vi "Signal in Single Point.vi"() -> ()   [LabVIEW 2025]
uses:
  <vilib>/xnet/xnet.llb/XNET Create Session (Signal Input Single-point).vi
  <vilib>/xnet/xnet.llb/XNET Read (Signal Single-point).vi
panel:
  out "Barra":dbl(graph)
  out "Abs":dbl(graph)
  in  "signal list":refnum<k21>[](array[refnum])
  in  "Wait":u32=200
  in  "stop":bool
  in  "interface":refnum<k21>="CAN1"
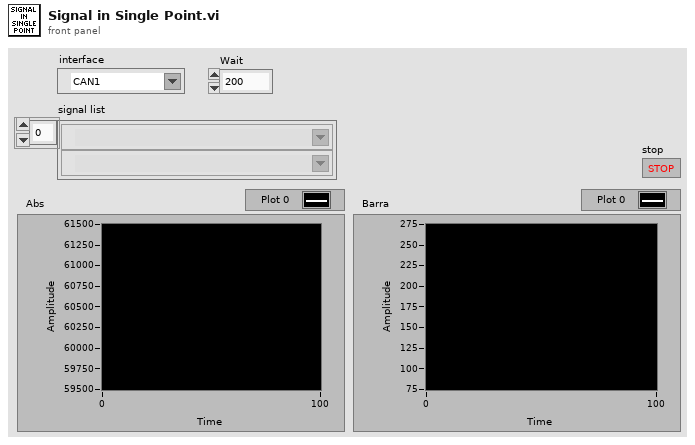
[diagram p1: front panel]
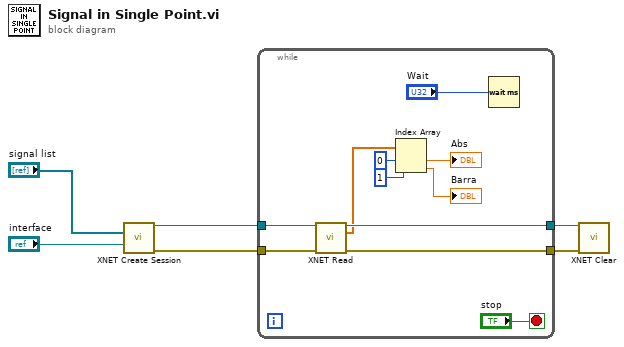
[diagram p0: block diagram]
diagram:
  n1 = call-poly <vilib>:"XNET Create Session.vi"("signal list"="signal list", "interface"="interface") -> ("session out"=w5:refnum<k21>, "error out"=w6:errorcluster)  [unwired: 12 in]
  n2 = while {
    tunnel: w6 -> [w16]
    tunnel: w5 -> [w17]
    tunnel: [w15] -> w3
    tunnel: [w14] -> w2
    stop <- "stop" stop-if-true
    n3 = call-poly <vilib>:"XNET Read.vi"("session in"=w17, "error in (no error)"=w16) -> ("session out"=w14:refnum<k21>, "data"=w11:dbl[], "error out"=w15:errorcluster)  [unwired: 11 in]
    n4 = Index Array(array=w11, index #1=0 ("index"), index #2=1 ("index")) -> (element #1=→"Abs":dbl, element #2=→"Barra":dbl)
    n5 = Wait (ms)(milliseconds to wait="Wait") -> ()  [unwired: 1 out]
  }
  n6 = call <vilib>:"XNET Clear.vi"("session in"=w2, "error in (no error)"=w3) -> ()  [unwired: 13 in, 1 out]
